vi "Run Substep by Index.vi"(8 "error in (no error)":errorcluster, 10 "Substep Index":i32, 11 "Step in":refnum<class "Step.lvclass">) -> (0 "error out":errorcluster, 2 "Change?":bool, 3 "Step out":refnum<class "Step.lvclass">)   [LabVIEW 2020, in "TSnax.lvlib" / "Step.lvclass"]
uses:
  Step.lvclass
  Step.lvclass/Step.ctl
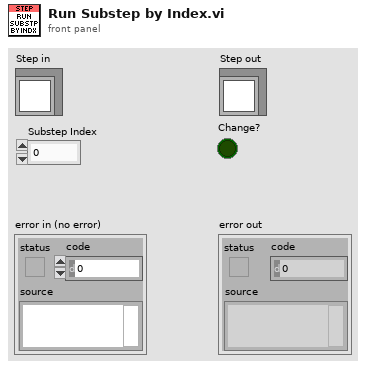
[diagram p1: front panel]
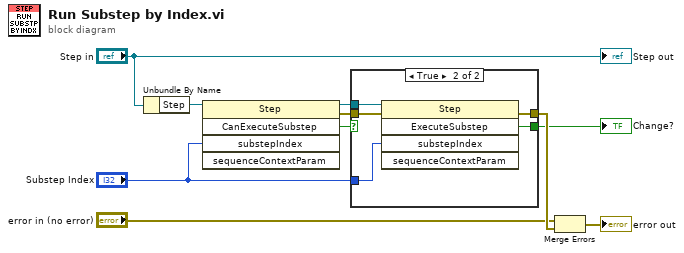
[diagram p0: block diagram]
diagram:
  n1 = Unbundle By Name("Step in") -> ("Step"=w5:refnum<k7>)
  n2 = invoke class="Step" method="CanExecuteSubstep"(reference=w5, "substepIndex"="Substep Index") -> (reference out=w9:refnum<k7>, error out=w8:errorcluster, "CanExecuteSubstep"=w7:bool)  [unwired: 3 in, 2 out]
  n3 = case shown="True" w7 {
    tunnel: w9 -> [_ w16]
    tunnel: w8 -> [w11 w15]
    tunnel: "Substep Index" -> [_ w14]
    tunnel: [_ w13] -> w3
    tunnel: [w11 w12] -> w10
    frame False {
    }
    frame True {
      n4 = invoke class="Step" method="ExecuteSubstep"(reference=w16, error in=w15, "substepIndex"=w14) -> (error out=w12:errorcluster, "ExecuteSubstep"=w13:bool)  [unwired: 2 in, 3 out]
    }
  }
  "Change?" <- w3
  n5 = Merge Errors("error in (no error)", w10) -> (→"error out":errorcluster)
  "Step out" <- "Step in"
